vi "TSM Fgen Initialize Sessions.vi"(0 "TSM context":T1) -> (15 "error out":errorcluster)   [LabVIEW 2020]
doc: "Use this VI to initialize sessions for all NI-FGEN instruments in the pin map associated with the test program."
uses:
  <vilib>/NI_TestStand_SemiconductorModule/NI_TestStand_Semiconductor_Module.lvlibp/PinMap/General/SemiconductorModuleContext.ctl
  <vilib>/NI_TestStand_SemiconductorModule/NI_TestStand_Semiconductor_Module.lvlibp
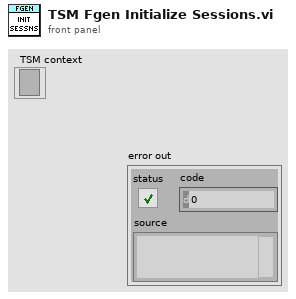
[diagram p1: front panel]
types:
  T1 = typedef "NI_TestStand_Semiconductor_Module.lvlibp/SemiconductorModuleContext.ctl" = refnum<k7>
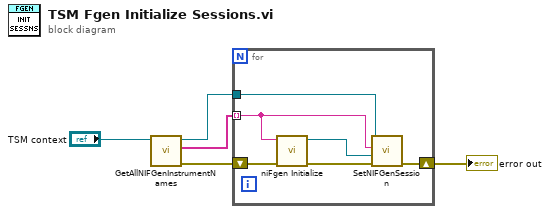
[diagram p0: block diagram]
diagram:
  n1 = call <vilib>:"GetAllNIFGenInstrumentNames.vi"("Semiconductor Module Context"="TSM context") -> ("error out"=w1:errorcluster, "Instrument Names"=w5:string[], "Semiconductor Module Context Out"=w4:T1)  [unwired: 8 in]
  n2 = for {
    tunnel: w5 -> [w9] mode=indexing
    tunnel: w4 -> [w7]
    shift-right: [w8] -> w2
    shift-left: w1 -> [w11]
    n3 = call <instrlib>:"niFgen Initialize.vi"("error in (no error)"=w11, "Resource Name"=w9) -> ("error out"=w10:errorcluster, "Instrument Handle Out"=w6:refnum<k15>)  [unwired: 8 in]
    n4 = call <vilib>:"SetNIFGenSession.vi"("error in (no error)"=w10, "Instrument Session"=w6, "Instrument Name"=w9, "Semiconductor Module Context"=w7) -> ("error out"=w8:errorcluster)  [unwired: 6 in, 1 out]
  }
  "error out" <- w2
